vi "Block List UI.vi"() -> ()   [LabVIEW 2022 SP3, in "FlexBlocks Support.lvlib"]
uses:
  FlexBlocks Support.lvlib
  <vilib>/regexp/Match Regular Expression.xnode
  <vilib>/IlluminatedG/IG AutoComplete/AutoComplete/AutoComplete.lvlib
panel:
  in  "SearchList":i32(listbox)
  in  "Collapse":bool
  in  "Refresh Workers":bool
  in  "New Block":bool
  in  "Blocks":string(tree)
  in  "Worker Search":string
  in  "Clear Search":bool
  out "Icon":picture
  out "Worker Name":string
  out "Desc":string
  in  "Open Block":bool
  in  "Values":string(tree)
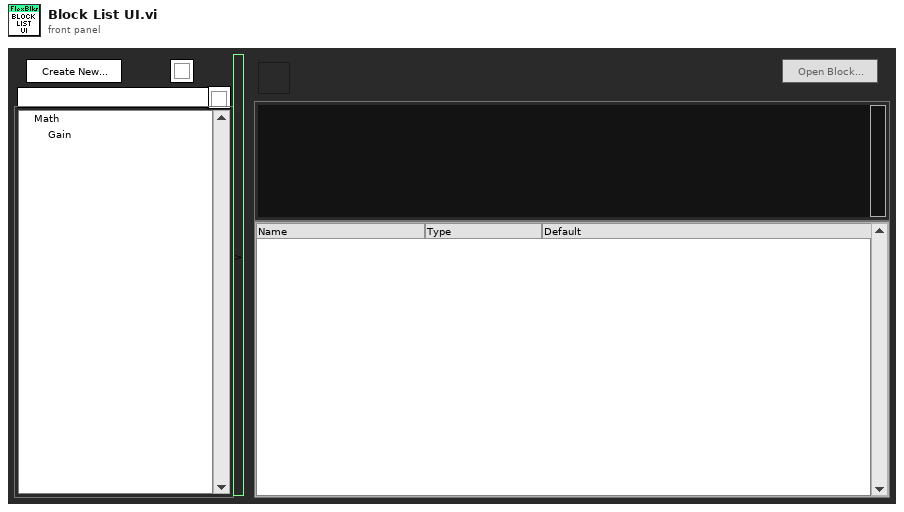
[diagram p1: front panel]
types:
  T1 = typedef "FlexBlocks Support.lvlib/UI State.ctl" = enum16{"Init", "Load", "Ready", "Run", "Cleanup", "Close"}
  T2 = enum32{"Invalid", "Standard", "Closed", "Hidden", "Minimized", "Maximized"}
  T3 = enum8{"Enabled", "Disabled", "Disabled and Grayed Out"}
  T4 = typedef "FlexBlocks Support.lvlib/New Block Config.ctl" = cluster{"Name":string, "Actions":T5, "IO Control":bool, "New Project?":bool, "Project":refnum<vi>}
  T5 = typedef "FlexBlocks Support.lvlib/Action Selections.ctl" = cluster{"Init":bool, "Start":bool, "Run":bool, "Stop":bool, "Close":bool}
  T6 = typedef "FlexBlocks Support.lvlib/Type Descriptor.ctl" = cluster{"Name":string, "Direction":T7, "Default":variant, "Min":variant, "Max":variant, "Step":variant, "Value Mode":T8, "Color":u32, "Options":string[], "Type String":string, "Item Path":path, "Required":bool, "Connpane Index":i32, "Special Terminal":T9, "Sort":i32}
  T7 = typedef "FlexBlocks Support.lvlib/Terminal Direction.ctl" = enum16{"Sink", "Source"}
  T8 = typedef "FlexBlocks Support.lvlib/Value Mode.ctl" = enum16{"Normal", "Range", "Select"}
  T9 = typedef "FlexBlocks Support.lvlib/Special Terminal.ctl" = enum16{"None", "Action", "Init", "Tag", "State in", "State out", "Error", "Control"}
  T10 = typedef "FlexBlocks Support.lvlib/Worker Info.ctl" = cluster{"Name":string, "Icon":T11, "Index":i32, "Variants":map{string, T12}, "Categories":string[]}
  T11 = typedef "imagedata.ctl" = cluster{"image type":i32, "image depth":i32, "image":u8[], "mask":u8[], "colors":u32[], "Rectangle":cluster{"left":i16, "top":i16, "right":i16, "bottom":i16}}
  T12 = typedef "FlexBlocks Support.lvlib/Worker Variant.ctl" = cluster{"Name":string, "Icon":T11}
  T13 = typedef "FlexBlocks Support.lvlib/Paths.ctl" = cluster{"FlexBlocks":path, "Workers Root":path, "Specialized Editors":path, "Worker Template":path, "SM Template":path, "Read Control Value Vim":path, "Write Indicator Value Vim":path, "XNode":path}
  T14 = typedef "LVRectTypeDef.ctl" = cluster{"Left":i16, "Top":i16, "Right":i16, "Bottom":i16}
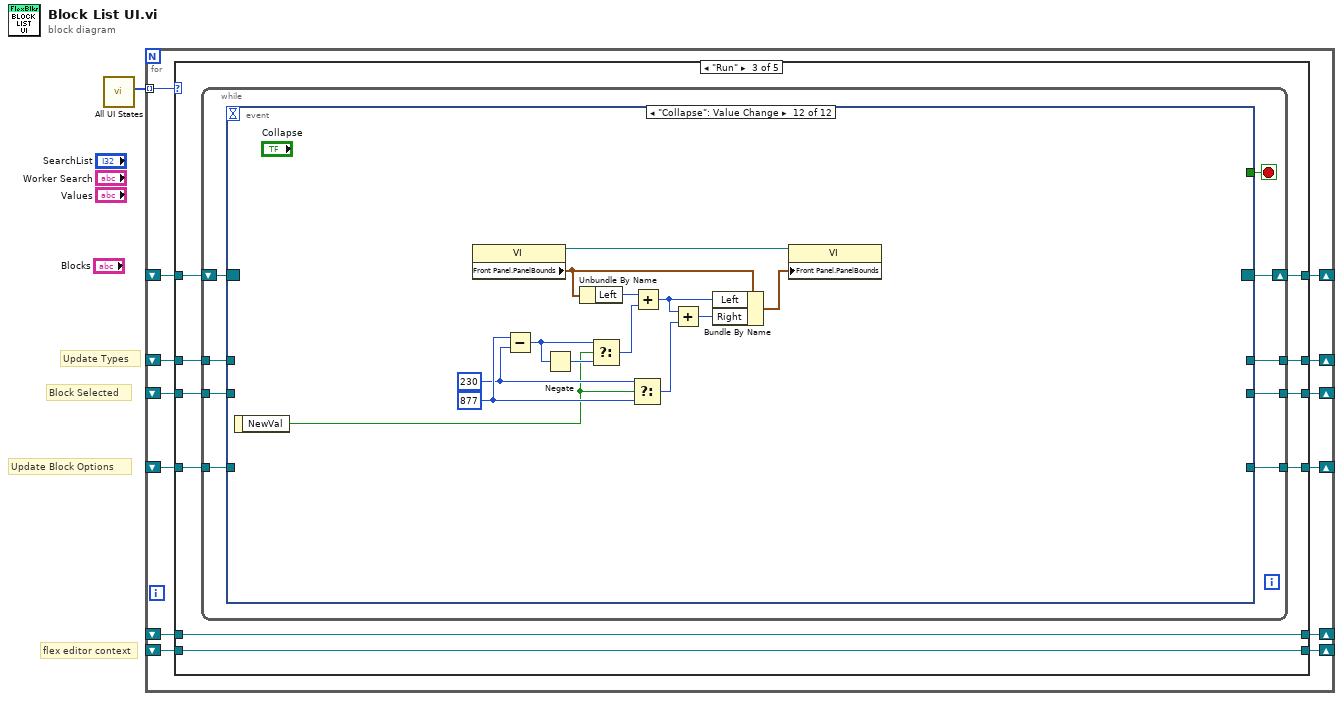
[diagram p0: block diagram]
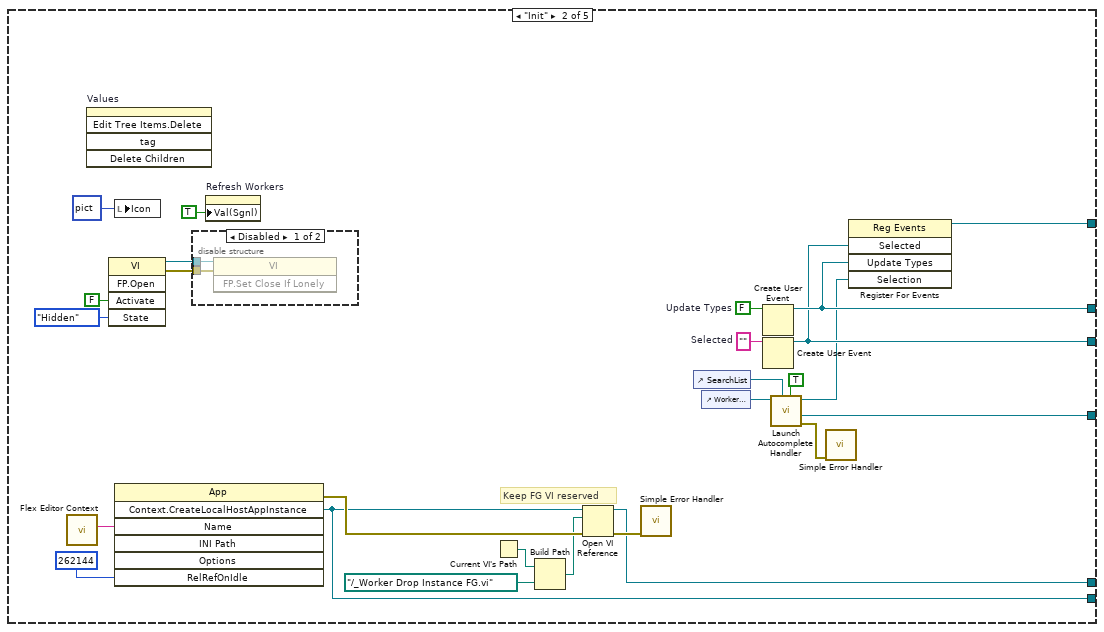
[diagram p3: hidden frame]
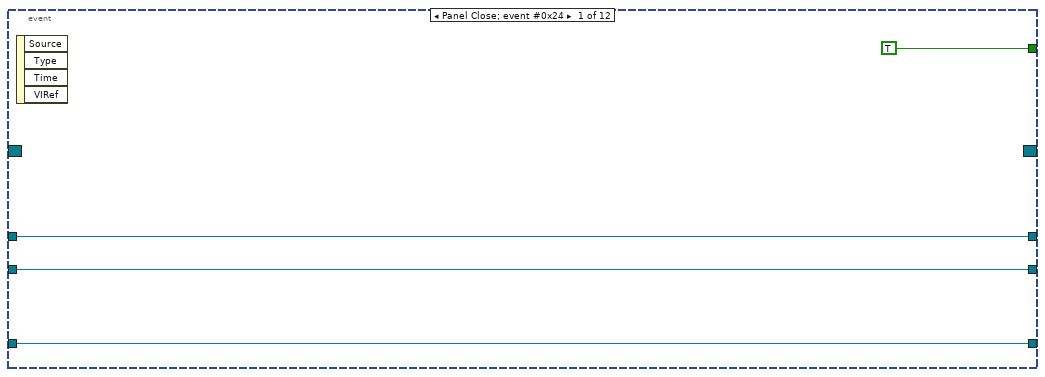
[diagram p5: hidden frame]
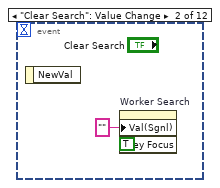
[diagram p6: hidden frame]
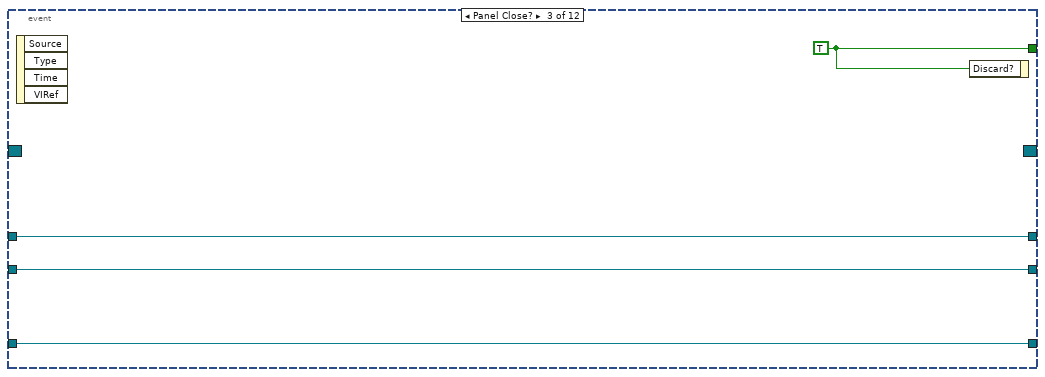
[diagram p7: hidden frame]
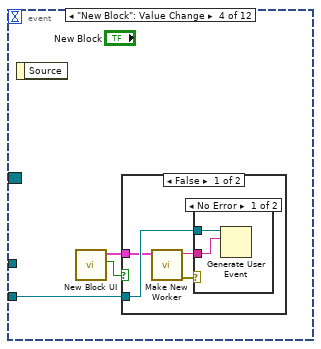
[diagram p8: hidden frame]
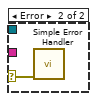
[diagram p9: hidden frame]
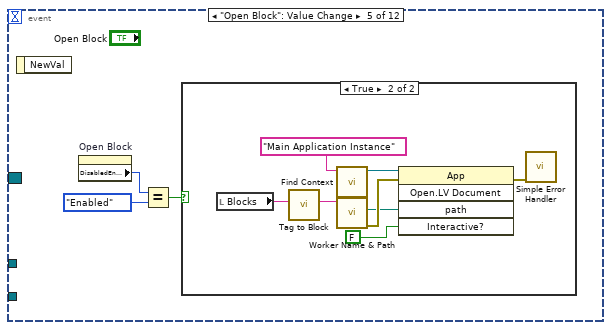
[diagram p11: hidden frame]
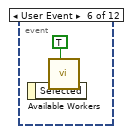
[diagram p13: hidden frame]
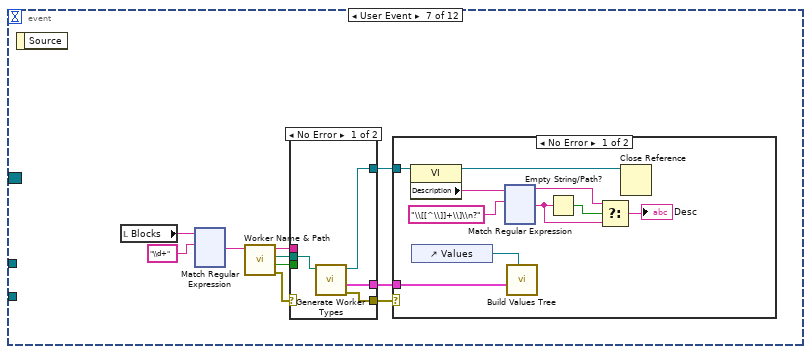
[diagram p14: hidden frame]
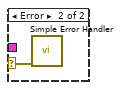
[diagram p15: hidden frame]
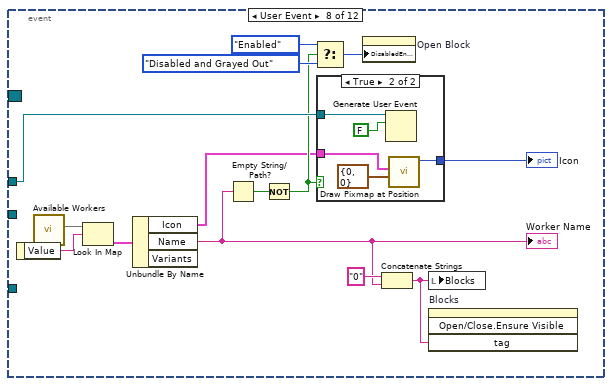
[diagram p17: hidden frame]
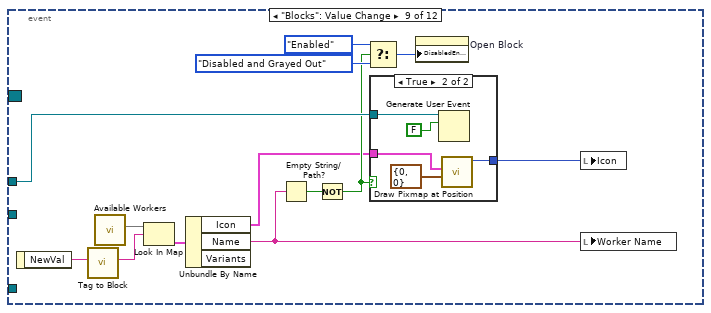
[diagram p19: hidden frame]
diagram:
  # "flex editor context"
  # "Update Block Options"
  # "Block Selected"
  # "Update Types"
  n1 = call "All UI States.vi"() -> ("All UI States"=w1:T1[])  [unwired: 11 in]
  n2 = for {
    tunnel: w1 -> [w14] mode=indexing
    shift-right: [w13] -> _
    shift-left: _ -> [w10]
    shift-right: [w12] -> _
    shift-left: _ -> [w9]
    shift-right: [w11] -> _
    shift-left: _ -> [w8]
    shift-right: [w7] -> _
    shift-left: _ -> [w6]
    shift-right: [w5] -> _
    shift-left: _ -> [w4]
    shift-right: [w3] -> _
    shift-left: _ -> [w2]
    n3 = case shown="\"Run\"" w14 {
      tunnel: [w20 w35 w57 refnum<event-registration> refnum ("Event Registration Refnum") w455] -> w13
      tunnel: [w19 w40 w54 refnum<user-event> refnum ("Update Types") w454] -> w12
      tunnel: [w18 w39 w53 refnum<user-event> refnum ("Selected") w453] -> w11
      tunnel: w10 -> [w20 _ w58 w449 w455]
      tunnel: w9 -> [w19 _ w56 w448 w454]
      tunnel: w8 -> [w18 _ w55 w447 w453]
      tunnel: [w17 w37 w51 refnum<user-event> refnum ("New Options Event") w452] -> w7
      tunnel: w6 -> [w17 _ w52 w444 w452]
      tunnel: [w16 w25 w50 refnum<vi> refnum ("Create Context") w451] -> w5
      tunnel: w4 -> [w16 _ w50 w438 w451]
      tunnel: [w15 w24 w49 refnum<vi> refnum ("vi reference") w450] -> w3
      tunnel: w2 -> [w15 _ w49 w440 w450]
      frame Default {
      }
      frame "Init" {
        w41 = FALSE  # Update Types
        w42 = ""  # Selected
        # "Keep FG VI reserved"
        n4 = call "Flex Editor Context.vi"() -> ("Flex Editor Context"=w30:string)  [unwired: 11 in]
        n5 = invoke on="Values" class="Tree (strict)" method="Edit Tree Items.Delete"() -> ()  [unwired: 5 in, 5 out]
        n6 = invoke class="VI" method="FP.Open"("Activate"=FALSE ("Activate?"), "State"=T2."Hidden") -> (reference out=w32:refnum<vi>, error out=w33:errorcluster)  [unwired: 3 in, 3 out]
        n7 = local write "Icon"(picture data[5B] ("empty picture")) -> ()
        n8 = invoke class="App" method="Context.CreateLocalHostAppInstance"("Name"=w30, "Options"=262144) -> (error out=w46:errorcluster, "Create Context"=w25:refnum<vi>)  [unwired: 5 in, 5 out]
        n9 = disable-structure shown="Disabled" {
          disable-tunnel: w33 -> [w48 _]
          disable-tunnel: w32 -> [w47 _]
          frame Disabled {
            n10 = invoke class="VI" method="FP.Set Close If Lonely"(reference=w47, error in=w48) -> ()  [unwired: 1 in, 3 out]
          }
          frame Enabled {
          }
        }
        n11 = property on="Refresh Workers" class="Bool (strict)"("Val(Sgnl)"=TRUE ("Value (Signaling)")) -> ()  [unwired: 2 in, 2 out]
        n12 = Current VI's Path() -> (path=w29:path)
        n13 = Build Path(base path=w29, name or relative path=path "../_Worker Drop Instance FG.vi") -> (appended path=w27:path)
        n14 = Open VI Reference(application reference (local)=w25, vi path=w27, error in (no error)=w46) -> (vi reference=w24:refnum<vi>, error out=w26:errorcluster)  [unwired: 3 in]
        n15 = call <vilib>:"Simple Error Handler.vi"("error in (no error)"=w26) -> ()  [unwired: 4 in, 5 out]
        n16 = control-ref of="SearchList"() -> (w22:refnum<vi>)
        n17 = control-ref of="Worker Search"() -> (w38:refnum<vi>)
        n18 = Create User Event(user event datatype=w41) -> (user event=w40:refnum<user-event>)  [unwired: 1 in, 1 out]
        n19 = Create User Event(user event datatype=w42) -> (user event=w39:refnum<user-event>)  [unwired: 1 in, 1 out]
        n20 = call <vilib>:"Launch Autocomplete Handler.vi"("Autohide ListBox (F)"=TRUE, "ListBox Refnum (Popup)"=w22, "Str Refnum"=w38) -> ("error out"=w23:errorcluster, "New Options Event"=w37:refnum<user-event>, "Selection"=w34:refnum<user-event>)  [unwired: 5 in, 1 out]
        n21 = call <vilib>:"Simple Error Handler.vi"("error in (no error)"=w23) -> ()  [unwired: 4 in, 5 out]
        n22 = register-events(w39, w40, w34) -> (reference out=w35:refnum<event-registration>)  [unwired: 2 in, 1 out]
      }
      frame "Run" {
        n23 = while {
          shift-right: [w60] -> w57
          shift-left: w58 -> [w61]
          tunnel: w56 -> [w66]
          tunnel: w55 -> [w65]
          tunnel: [w64] -> w54
          tunnel: [w63] -> w53
          tunnel: w52 -> [w62]
          tunnel: [w59] -> w51
          stop <- w67 stop-if-true
          n24 = event shown="[11] \"Collapse\": Value Change" {
            selector: w61 -> [_ _ _ _ _ _ _ _ _ _ _ _]
            dyn-events: [_ _ _ _ _ _ _ _ _ _ _ _] -> w60
            timeout: _ -> [_ _ _ _ _ _ _ _ _ _ _ _]
            tunnel: [TRUE ("Discard?") _ w77 _ _ _ _ _ _ _ _ _] -> w67
            tunnel: w66 -> [w70 _ w76 _ _ _ _ w372 w391 _ _ _]
            tunnel: w65 -> [w69 _ w75 w79 _ _ _ _ _ _ _ _]
            tunnel: [w70 _ w76 _ _ _ _ _ _ _ _ _] -> w64
            tunnel: [w69 _ w75 _ _ _ _ _ _ _ _ _] -> w63
            tunnel: w62 -> [w68 _ w74 _ _ _ _ _ _ w410 _ _]
            tunnel: [w68 _ w74 _ _ _ _ _ _ _ _ _] -> w59
            event Panel Close; event #0x24 {
              n25 = event-data() -> ()  [unwired: 1 in, 4 out]
            }
            event "Clear Search": Value Change {
              n26 = event-data() -> ()  [unwired: 1 in, 1 out]
              n27 = property on="Worker Search" class="Str"("Val(Sgnl)"="" ("Value (Signaling)"), "Key Focus"=TRUE) -> ()  [unwired: 2 in, 2 out]
            }
            event Panel Close? {
              w77 = TRUE ("Discard?")
              n28 = event-data() -> ()  [unwired: 1 in, 4 out]
              n29 = event-data("Discard?"=w77) -> ()  [unwired: 1 in, 1 out]
            }
            event "New Block": Value Change {
              n30 = event-data() -> ()  [unwired: 1 in, 1 out]
              n31 = call "New Block UI.vi"() -> ("Cancelled?"=w80:bool, "New Block Config"=w78:T4)  [unwired: 10 in]
              n32 = case shown="False" w80 {
                tunnel: w79 -> [w84 _]
                tunnel: w78 -> [w82 _]
                frame False {
                  n33 = call "Make New Worker.vi"("New Block Config"=w82) -> ("error out"=w83:errorcluster, "Block Name"=w81:string)  [unwired: 9 in]
                  n34 = case shown="No Error" w83 {
                    selector: w83 -> [_ w87]
                    tunnel: w84 -> [w86 _]
                    tunnel: w81 -> [w85 _]
                    frame No Error {
                      n35 = Generate User Event(user event=w86, event data cluster=w85) -> ()  [unwired: 2 in, 2 out]
                    }
                    frame Error {
                      n36 = call <vilib>:"Simple Error Handler.vi"("error in (no error)"=w87) -> ()  [unwired: 4 in, 5 out]
                    }
                  }
                }
                frame True {
                }
              }
            }
            event "Open Block": Value Change {
              n37 = event-data() -> ()  [unwired: 1 in, 1 out]
              n38 = property on="Open Block" class="Bool"() -> ("DisabledEnum"=w90:T3)  [unwired: 2 in, 2 out]
              n39 = Equal?(x=w90, y=T3."Enabled") -> (x = y?=w88:bool)
              n40 = case shown="True" w88 {
                frame False {
                }
                frame True {
                  n41 = local read "Blocks"() -> (w92:string)
                  n42 = call "Tag to Block.vi"("Block Tag"=w92) -> ("Block"=w91:string)  [unwired: 10 in]
                  n43 = call "Find Context.vi"("Name"="Main Application Instance") -> ("App"=w94:refnum<vi>)  [unwired: 9 in, 1 out]
                  n44 = call "Worker Name & Path.vi"("Worker"=w91) -> ("error out"=w98:errorcluster, "lvlib Path"=w97:path)  [unwired: 6 in, 3 out]
                  n45 = invoke class="App" method="Open.LV Document"(reference=w94, error in=w98, "path"=w97, "Interactive?"=FALSE) -> (error out=w95:errorcluster)  [unwired: 1 in, 4 out]
                  n46 = call <vilib>:"Simple Error Handler.vi"("error in (no error)"=w95) -> ()  [unwired: 4 in, 5 out]
                }
              }
            }
            event User Event {
              n47 = event-data() -> ()  [unwired: 1 in, 1 out]
              n48 = call "Available Workers.vi"("Refresh? (F)"=TRUE) -> ()  [unwired: 9 in, 2 out]
            }
            event User Event {
              n49 = event-data() -> ()  [unwired: 1 in, 1 out]
              n50 = local read "Blocks"() -> (w102:string)
              n51 = xnode "Match Regular Expression"("input string"=w102, "regular expression"="\\d+") -> ("after match"=w100:string)  [unwired: 4 in, 4 out]
              n52 = call "Worker Name & Path.vi"("Worker"=w100) -> ("error out"=w109:errorcluster, "Is Worker Variant"=w108:bool, "lvlib Path"=w107:path, "Display Name"=w106:string)  [unwired: 6 in, 1 out]
              n53 = case shown="No Error" w109 {
                selector: w109 -> [_ w359]
                tunnel: w108 -> [_ _]
                tunnel: w107 -> [w357 _]
                tunnel: w106 -> [_ _]
                tunnel: [w358 w359] -> w105
                tunnel: [w356 _] -> w104
                tunnel: [w355 _] -> w103
                frame No Error {
                  n54 = call "Generate Worker Types.vi"("Worker lvlib"=w357) -> ("error out"=w358:errorcluster, "Types"=w356:T6[], "Worker VI"=w355:refnum<vi>)  [unwired: 7 in, 1 out]
                }
                frame Error {
                }
              }
              n55 = case shown="No Error" w105 {
                selector: w105 -> [_ w354]
                tunnel: w104 -> [w236 _]
                tunnel: w103 -> [w234 _]
                frame No Error {
                  n56 = property class="VI"(reference=w234) -> (reference out=w233:refnum<vi>, "Description"=w232:string)  [unwired: 1 in, 1 out]
                  n57 = control-ref of="Values"() -> (w235:refnum<vi>)
                  n58 = xnode "Match Regular Expression"("input string"=w232, "regular expression"="\\[[^\\]]+\\]\\n?") -> ("before match"=w229:string, "after match"=w228:string)  [unwired: 4 in, 3 out]
                  n59 = call "Build Values Tree.vi"("Tree"=w235, "Types"=w236) -> ()  [unwired: 10 in]
                  n60 = Empty String/Path?(string/path=w228) -> (empty?=w230:bool)
                  n61 = Select(t=w229, s=w230, f=w228) -> (s? t:f=→"Desc":string)
                  n62 = Close Reference(reference=w233) -> ()  [unwired: 1 in, 1 out]
                }
                frame Error {
                  n63 = call <vilib>:"Simple Error Handler.vi"("error in (no error)"=w354) -> ()  [unwired: 4 in, 5 out]
                }
              }
            }
            event User Event {
              n64 = event-data() -> ("Value"=w373:string)  [unwired: 1 in]
              n65 = call "Available Workers.vi"() -> ("Workers Map"=w365:map{string, T10})  [unwired: 10 in, 1 out]
              n66 = Look In Map(map=w365, key=w373) -> (value=w364:T10)  [unwired: 1 in, 1 out]
              n67 = Unbundle By Name(w364) -> ("Icon"=w367:T11, "Name"=w361:string)  [unwired: 1 out]
              "Worker Name" <- w361
              n68 = Empty String/Path?(string/path=w361) -> (empty?=w371:bool)
              n69 = Not(x=w371) -> (.not. x?=w368:bool)
              n70 = Select(t=T3."Enabled" ("Disabled"), s=w368, f=T3."Disabled and Grayed Out" ("Disabled")) -> (s? t:f=w363:T3)
              n71 = case shown="True" w368 {
                tunnel: w372 -> [_ w378]
                tunnel: w367 -> [_ w375]
                tunnel: [_ w374] -> w366
                frame False {
                }
                frame True {
                  n72 = Generate User Event(user event=w378, event data cluster=FALSE ("event data")) -> ()  [unwired: 2 in, 2 out]
                  n73 = call "Draw Pixmap at Position.vi"("Position"=cluster{"left":i16, "top":i16} {"left"=0, "top"=0}, "Pixmap"=w375) -> ("2D Picture"=w374:picture)  [unwired: 9 in]
                }
              }
              "Icon" <- w366
              n74 = property on="Open Block" class="Bool"("DisabledEnum"=w363) -> ()  [unwired: 2 in, 2 out]
              n75 = Concatenate Strings("0" ("string"), w361) -> (w360:string)
              n76 = local write "Blocks"(w360) -> ()
              n77 = invoke on="Blocks" class="Tree (strict)" method="Open/Close.Ensure Visible"("tag"=w360) -> ()  [unwired: 3 in, 4 out]
            }
            event "Blocks": Value Change {
              n78 = event-data() -> ("NewVal"=w380:string)  [unwired: 1 in]
              n79 = call "Tag to Block.vi"("Block Tag"=w380) -> ("Block"=w379:string)  [unwired: 10 in]
              n80 = call "Available Workers.vi"() -> ("Workers Map"=w385:map{string, T10})  [unwired: 10 in, 1 out]
              n81 = Look In Map(map=w385, key=w379) -> (value=w384:T10)  [unwired: 1 in, 1 out]
              n82 = Unbundle By Name(w384) -> ("Icon"=w386:T11, "Name"=w381:string)  [unwired: 1 out]
              n83 = Empty String/Path?(string/path=w381) -> (empty?=w390:bool)
              n84 = Not(x=w390) -> (.not. x?=w387:bool)
              n85 = Select(t=T3."Enabled" ("Disabled"), s=w387, f=T3."Disabled and Grayed Out" ("Disabled")) -> (s? t:f=w383:T3)
              n86 = case shown="True" w387 {
                tunnel: w391 -> [_ w396]
                tunnel: w386 -> [_ w393]
                tunnel: [_ w392] -> w382
                frame False {
                }
                frame True {
                  n87 = Generate User Event(user event=w396, event data cluster=FALSE ("event data")) -> ()  [unwired: 2 in, 2 out]
                  n88 = call "Draw Pixmap at Position.vi"("Position"=cluster{"left":i16, "top":i16} {"left"=0, "top"=0}, "Pixmap"=w393) -> ("2D Picture"=w392:picture)  [unwired: 9 in]
                }
              }
              n89 = property on="Open Block" class="Bool"("DisabledEnum"=w383) -> ()  [unwired: 2 in, 2 out]
              n90 = local write "Icon"(w382) -> ()
              n91 = local write "Worker Name"(w381) -> ()
            }
            event "Refresh Workers": Value Change {
              w406 = T3."Disabled and Grayed Out" ("Disabled")
              # "Clear out search text to prevent filtering after refreshing."
              n92 = event-data() -> ()  [unwired: 1 in, 1 out]
              n93 = invoke on="Blocks" class="Tree (strict)" method="Edit Tree Items.Delete"() -> (error out=w405:errorcluster)  [unwired: 5 in, 4 out]
              n94 = local write "Refresh Workers"(FALSE ("Refresh Workers")) -> ()
              n95 = property on="Worker Search" class="Str"("DisabledEnum"=w406) -> ()  [unwired: 2 in, 2 out]
              n96 = property on="Clear Search" class="Bool"("DisabledEnum"=w406) -> ()  [unwired: 2 in, 2 out]
              n97 = property on="Open Block" class="Bool"("DisabledEnum"=w406) -> ()  [unwired: 2 in, 2 out]
              n98 = invoke on="Blocks" class="Tree (strict)" method="Edit Tree Items.Add Item to End"(error in=w405, "Left Cell"="Identifying Workers...", "Child Only?"=FALSE) -> (error out=w402:errorcluster)  [unwired: 5 in, 7 out]
              n99 = control-ref of="Blocks"() -> (w401:refnum<vi>)
              n100 = call "Available Workers.vi"("Refresh? (F)"=TRUE) -> ("Workers Map"=w398:map{string, T10}, "Names"=w400:string[])  [unwired: 9 in]
              n101 = call "Build Blocks Tree.vi"("error in (no error)"=w402, "Blocks Map"=w398, "Blocks Tree"=w401) -> ("error out"=w399:errorcluster)  [unwired: 8 in]
              n102 = property on="Worker Search" class="Str"(error in=w399, "Text.Text"="") -> (error out=w407:errorcluster)  [unwired: 1 in, 1 out]
              n103 = invoke class="VI" method="FP.Open"(error in=w407, "Activate"=TRUE ("Activate?"), "State"=T2."Standard") -> (error out=w397:errorcluster)  [unwired: 2 in, 4 out]
              n104 = Generate User Event(user event=w410, event data cluster=w400, error in=w397) -> (error out=w409:errorcluster)  [unwired: 1 in, 1 out]
              n105 = call <vilib>:"Simple Error Handler.vi"("error in (no error)"=w397) -> ()  [unwired: 4 in, 5 out]
              n106 = flat-sequence {
                tunnel: w409 -> [_]
                frame #0 {
                  w415 = T3."Enabled" ("Disabled")
                  n107 = property on="Worker Search" class="Str"("DisabledEnum"=w415) -> ()  [unwired: 2 in, 2 out]
                  n108 = property on="Clear Search" class="Bool"("DisabledEnum"=w415) -> ()  [unwired: 2 in, 2 out]
                }
              }
            }
            event "Blocks": Drag Starting? {
              n109 = event-data() -> ()  [unwired: 1 in, 2 out]
              n110 = local read "Blocks"() -> (w416:string)
              n111 = call "Tag to Block.vi"("Block Tag"=w416) -> ("Block"=w417:string)  [unwired: 10 in]
              n112 = call "Paths.vi"() -> ("Paths"=w420:T13)  [unwired: 11 in]
              n113 = call "Worker Name & Path.vi"("Worker"=w417) -> ("lvlib Path"=w422:path)  [unwired: 6 in, 4 out]
              n114 = Unbundle By Name(w420) -> ("XNode"=w419:path)
              n115 = call "Call Worker Drop Instance.vi"("Worker Path In"=w422) -> ("error out"=w421:errorcluster)  [unwired: 9 in, 1 out]
              n116 = invoke class="App" method="UI.PlaceObjectOnCursor"(error in=w421, "path"=w419) -> (error out=w418:errorcluster)  [unwired: 4 in, 5 out]
              n117 = call <vilib>:"Simple Error Handler.vi"("error in (no error)"=w418) -> ()  [unwired: 4 in, 5 out]
              n118 = event-data("Discard?"=TRUE) -> ()  [unwired: 3 in, 1 out]
            }
            event "Collapse": Value Change {
              w432 = i16 877 ("y")
              w431 = i16 230 ("y")
              n119 = event-data() -> ("NewVal"=w428:bool)  [unwired: 1 in]
              n120 = property class="VI"() -> (reference out=w435:refnum<vi>, "Front Panel.PanelBounds"=w434:T14)  [unwired: 2 in, 1 out]
              n121 = Subtract(x=w432, y=w431) -> (x-y=w430:i16)
              n122 = Negate(x=w430) -> (-x=w429:i16)
              n123 = Unbundle By Name(w434) -> ("Left"=w433:i16)
              n124 = Select(t=w430, s=w428, f=w429) -> (s? t:f=w427:i16)
              n125 = Select(t=w431, s=w428, f=w432) -> (s? t:f=w424:i16)
              n126 = Add(x=w433, y=w427) -> (x+y=w425:i16)
              n127 = Add(x=w425, y=w424) -> (x+y=w426:i16)
              n128 = Bundle By Name(cluster=w434, "Left"=w425, "Right"=w426) -> (w436:T14)
              n129 = property class="VI"(reference=w435, "Front Panel.PanelBounds"=w436) -> ()  [unwired: 1 in, 2 out]
            }
          }
        }
      }
      frame "Cleanup" {
        n130 = Close Reference(reference=w440) -> (error out=w439:errorcluster)  [unwired: 1 in]
        n131 = Unregister For Events(event registration refnum=w449) -> ()  [unwired: 1 in, 1 out]
        n132 = Destroy User Event(user event=w448) -> ()  [unwired: 1 in, 1 out]
        n133 = Destroy User Event(user event=w447) -> ()  [unwired: 1 in, 1 out]
        n134 = Destroy User Event(user event=w444) -> ()  [unwired: 1 in, 1 out]
        n135 = Close Reference(reference=w438, error in (no error)=w439) -> ()  [unwired: 1 out]
      }
      frame "Close" {
        n136 = invoke class="VI" method="FP.Close"() -> ()  [unwired: 3 in, 3 out]
      }
    }
  }
